vi "Cross Term.vi"() -> ()   [LabVIEW 2023]
doc: "This example shows the concept of crossterms in the Wigner-Ville distribution (WVD). The WVD has the best joint time-frequency resolution among all known quadratic JTFA methods. However, the severe crossterm interference from a multi-component signal degrades the readability of the time-frequency representation and limits the extensive applications. \n\nCrossterms are artifacts that appear in the WVD representation between valid signal components or autoterms. These crossterms falsely indicate the existence of signal components between valid signal components.\n\n<b>Instructions:</b>\n1) Run this VI.\n2) Compare the spectrogram of the three signals to understand what autoterms and crossterms are in the time-frequency representation.\n3) Double-click the Time Frequency Spectrogram Express VI wired to the <b>Signal A + Signal B</b> indicator on the Block Diagram of this example to investigate the crossterms of other TFA methods."
uses:
  Instance           3 18Saved   Cross Term .vi
  Instance           2 18Saved   Cross Term .vi
  Instance           4 18Saved   Cross Term .vi
  <vilib>/addons/Time Frequency Analysis/_control.llb/TFA Configure Spectrogram Indicator (Predefined Color Table).vi
  <vilib>/addons/_Advanced Signal Processing/NI_AdvSigProcTFA.lvlib
panel:
  out "WVD of Signal A + Signal B":dbl[][](graph)
  out "Signal A + Signal B":dbl[](graph)
  out "WVD of Signal B":dbl[][](graph)
  out "Signal B":dbl[](graph)
  out "Signal A":dbl[](graph)
  out "WVD of Signal A":dbl[][](graph)
  # "Overview: Shows the concept of crossterms in the Wigner-Ville distribution (WVD). \nRequirements: LabVIEW Full Development System, Advanced Signal Processing Toolkit\nInstructions: \n1. Run this VI.\n2. Compare the spectrogram of the three signals to understand what auto terms and cross terms are in the time-frequency representation.\n3. Double-click the Time Frequency Spectrogram Express VI wired to the Signal A + Signal B indicator on the block diagram of this example to investigate the cross terms of other TFA methods."
  # "Cross term"
  # "Auto terms"
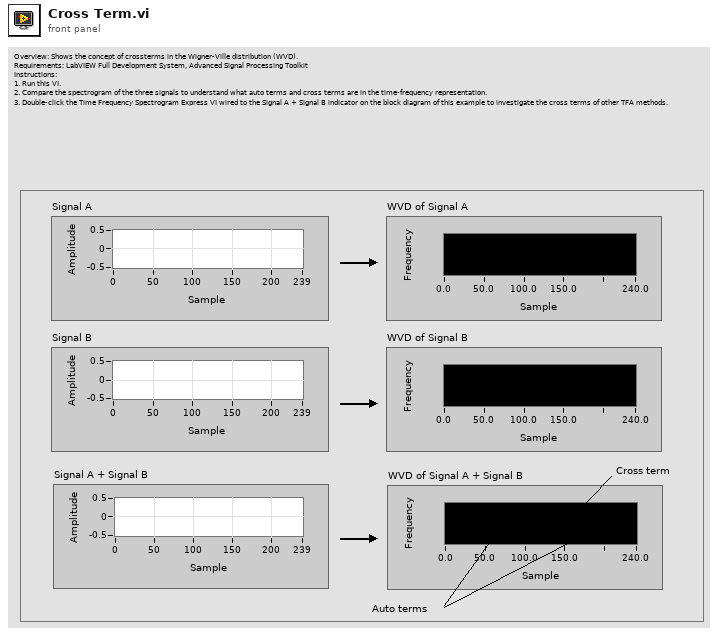
[diagram p1: front panel]
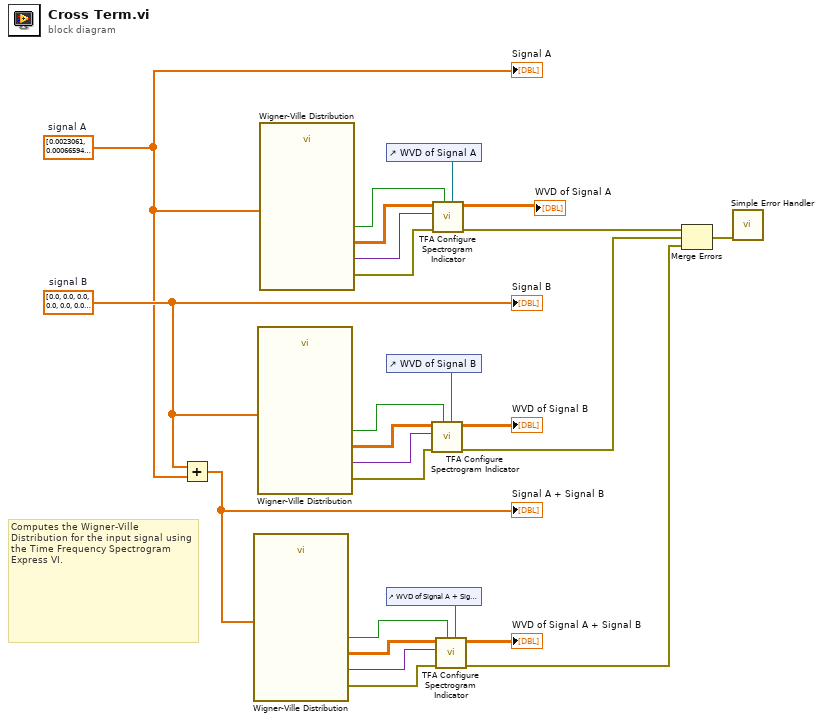
[diagram p0: block diagram]
diagram:
  w9 = dbl[] [0.0023061, 0.00066594, -0.00077047, -0.0011251, -0.00086556, -0.00060952, -2.9219e-06, 0.00096374, 0.00093837, -0.0003896, -0.00080533, 0.00055482, 0.00077422, -0.0012548, -0.001366, 0.0018099, 0.0021158, -0.0023846, -0.0028825, 0.0033362, 0.0039461, -0.0046839, -0.0054606, 0.0063973, 0.0074343, -0.0086009, -0.0099485, 0.011453, 0.013156, -0.015069, -0.017196, 0.019567, 0.022191, -0.025087, -0.028275, 0.031766, 0.035577, -0.039721, -0.044206, 0.049045, 0.054241, -0.0598, -0.065721, 0.072002, 0.078634, -0.085609, -0.092908, 0.10051, 0.1084, -0.11654, -0.12489, 0.13342, 0.14209, -0.15085, -0.15964, 0.16842, 0.17711, -0.18567, -0.19404, 0.20214, 0.20992, -0.21732, -0.22426, 0.23071, 0.23659, -0.24186, -0.24647, 0.25038, 0.25355, -0.25596, -0.25757, 0.25838, 0.25838, -0.25757, -0.25596, 0.25355, 0.25038, -0.24647, -0.24186, 0.23659, 0.23071, -0.22426, -0.21732, 0.20992, 0.20214, -0.19404, -0.18567, 0.17711, 0.16842, -0.15964, -0.15085, 0.14209, 0.13342, -0.12489, -0.11654, 0.1084, 0.10051, -0.092908, -0.085609, 0.078635, 0.072002, -0.065721, -0.0598, 0.054241, 0.049045, -0.044207, -0.039721, 0.035578, 0.031767, -0.028275, -0.025088, 0.02219, 0.019565, -0.017197, -0.015067, 0.01316, 0.011458, -0.0099453, -0.0086049, 0.0074217, 0.0063812, -0.0054692, -0.0046729, 0.00398, 0.0033791, -0.00286, -0.002413, 0.0020295, 0.0017015, -0.0014221, -0.0011848, 0.00098404, 0.00081471, -0.0006724, -0.00055321, 0.00045371, 0.0, 0.0, 0.0, 0.0, 0.0, 0.0, 0.0, 0.0, 0.0, 0.0, 0.0, 0.0, 0.0, 0.0, 0.0, 0.0, 0.0, 0.0, 0.0, 0.0, 0.0, 0.0, 0.0, 0.0, 0.0, 0.0, 0.0, 0.0, 0.0, 0.0, 0.0, 0.0, 0.0, 0.0, 0.0, 0.0, 0.0, 0.0, 0.0, 0.0, 0.0, 0.0, 0.0, 0.0, 0.0, 0.0, 0.0, 0.0, 0.0, 0.0, 0.0, 0.0, 0.0, 0.0, 0.0, 0.0, 0.0, 0.0, 0.0, 0.0, 0.0, 0.0, 0.0, 0.0, 0.0, 0.0, 0.0, 0.0, 0.0, 0.0, 0.0, 0.0, 0.0, 0.0, 0.0, 0.0, 0.0, 0.0, 0.0, 0.0, 0.0, 0.0, 0.0, 0.0, 0.0, 0.0, 0.0, 0.0, 0.0, 0.0, 0.0, 0.0, 0.0, 0.0, 0.0, 0.0, 0.0, 0.0, 0.0, 0.0, 0.0, 0.0, 0.0, 0.0]  # signal A
  w17 = dbl[] [0.0, 0.0, 0.0, 0.0, 0.0, 0.0, 0.0, 0.0, 0.0, 0.0, 0.0, 0.0, 0.0, 0.0, 0.0, 0.0, 0.0, 0.0, 0.0, 0.0, 0.0, 0.0, 0.0, 0.0, 0.0, 0.0, 0.0, 0.0, 0.0, 0.0, 0.0, 0.0, 0.0, 0.0, 0.0, 0.0, 0.0, 0.0, 0.0, 0.0, 0.0, 0.0, 0.0, 0.0, 0.0, 0.0, 0.0, 0.0, 0.0, 0.0, 0.0, 0.0, 0.0, 0.0, 0.0, 0.0, 0.0, 0.0, 0.0, 0.0, 0.0, 0.0, 0.0, 0.0, 0.0, 0.0, 0.0, 0.0, 0.0, 0.0, 0.0, 0.0, 0.0, 0.0, 0.0, 0.0, 0.0, 0.0, 0.0, 0.0, 0.0, 0.0, 0.0, 0.0, 0.0, 0.0, 0.0, 0.0, 0.0, 0.0, 0.0, 0.0, 0.0, 0.0, 0.0, 0.0, 0.0, 0.0, 0.0, 0.0, 0.0, 0.0, 0.0, 0.0, 0.0, 0.0, 0.0, 0.0, 0.0, 0.0, 0.0, 0.0, 0.0, 0.0, 0.0, 0.0, 0.0, 0.0, 0.0, 0.0, 0.0005928, 0.00029939, -0.0003639, -0.0010645, -0.0012857, -0.00064123, 0.00076964, 0.0022232, 0.0026516, 0.0013059, -0.0015478, -0.004415, -0.0052001, -0.0025289, 0.0029599, 0.0083374, 0.009697, 0.0046569, -0.0053824, -0.014971, -0.017195, -0.0081544, 0.0093068, 0.025563, 0.028993, 0.013577, -0.015302, -0.041505, -0.046484, -0.021497, 0.023924, 0.06408, 0.07087, 0.032363, -0.035568, -0.094075, -0.10274, -0.046331, 0.050282, 0.13133, 0.14163, 0.063069, -0.067591, -0.17433, -0.18565, -0.081639, 0.086397, 0.22004, 0.23141, 0.10049, -0.10501, -0.26411, -0.27428, -0.11761, 0.12137, 0.30143, 0.30912, 0.13089, -0.13339, -0.32714, -0.33128, -0.13852, 0.1394, 0.3376, 0.3376, 0.1394, -0.13852, -0.33128, -0.32714, -0.13339, 0.13089, 0.30912, 0.30143, 0.12137, -0.11761, -0.27428, -0.26411, -0.10501, 0.10049, 0.23141, 0.22004, 0.086397, -0.081639, -0.18565, -0.17433, -0.067591, 0.063069, 0.14163, 0.13133, 0.050282, -0.046331, -0.10274, -0.094075, -0.035568, 0.032363, 0.07087, 0.06408, 0.023924, -0.021497, -0.046484, -0.041505, -0.015303, 0.013577, 0.028994, 0.025565, 0.0093048, -0.008157, -0.017191, -0.014967, -0.0053881, 0.0046495, 0.0097066, 0.0083498, 0.002944, -0.0025493, -0.0051742, -0.0043822, -0.0015894, 0.0012534, 0.0027177]  # signal B
  # "Computes the Wigner-Ville Distribution for the input signal using the Time Frequency Spectrogram Express VI."
  n1 = Add(x=w17, y=w9) -> (x+y=w16:dbl[])
  "Signal A + Signal B" <- w16
  n2 = call "Wigner-Ville Distribution"("Signal"=w16) -> ("error out"=w6:errorcluster, "Scale Info"=w10:variant, "Spectrogram"=w11:dbl[][], "dB"=w12:bool)  [unwired: 2 in, 5 out]
  n3 = call "Wigner-Ville Distribution"("Signal"=w17) -> ("error out"=w7:errorcluster, "Scale Info"=w14:variant, "Spectrogram"=w15:dbl[][], "dB"=w13:bool)  [unwired: 2 in, 5 out]
  n4 = call "Wigner-Ville Distribution"("Signal"=w9) -> ("error out"=w8:errorcluster, "Scale Info"=w19:variant, "Spectrogram"=w20:dbl[][], "dB"=w18:bool)  [unwired: 2 in, 5 out]
  n5 = control-ref of="WVD of Signal A"() -> (w25:refnum<vi>)
  n6 = control-ref of="WVD of Signal B"() -> (w24:refnum<vi>)
  n7 = control-ref of="WVD of Signal A + Signal B"() -> (w22:refnum<vi>)
  n8 = call-poly <vilib>:"TFA Configure Spectrogram Indicator.vi"("reference of TF spectrogram indicator"=w24, "dB on? (F)"=w13, "error in (no error)"=w7, "scale info"=w14, "spectrogram"=w15) -> ("error out"=w4:errorcluster, "TF spectrogram indicator"=→"WVD of Signal B":dbl[][])  [unwired: 2 in, 3 out]
  n9 = call-poly <vilib>:"TFA Configure Spectrogram Indicator.vi"("reference of TF spectrogram indicator"=w25, "dB on? (F)"=w18, "error in (no error)"=w8, "scale info"=w19, "spectrogram"=w20) -> ("error out"=w5:errorcluster, "TF spectrogram indicator"=→"WVD of Signal A":dbl[][])  [unwired: 2 in, 3 out]
  n10 = call-poly <vilib>:"TFA Configure Spectrogram Indicator.vi"("reference of TF spectrogram indicator"=w22, "dB on? (F)"=w12, "error in (no error)"=w6, "scale info"=w10, "spectrogram"=w11) -> ("error out"=w3:errorcluster, "TF spectrogram indicator"=→"WVD of Signal A + Signal B":dbl[][])  [unwired: 2 in, 3 out]
  n11 = Merge Errors(w5, w4, w3) -> (w2:errorcluster)
  n12 = call <vilib>:"Simple Error Handler.vi"("error in (no error)"=w2) -> ()  [unwired: 4 in, 5 out]
  "Signal A" <- w9
  "Signal B" <- w17
